vi "Read Power Meter Reverse.vi"(11 "AM-AM in":refnum<class "AM-AM.lvclass">) -> (2 "Power Meter.lvclass":refnum<class "Power Meter.lvclass">, 3 "AM-AM out":refnum<class "AM-AM.lvclass">)   [LabVIEW 2020, in "AM-AM.lvclass"]
uses:
  AM-AM.lvclass
  Instruments/Power Meter/Power Meter.lvclass
  AM-AM.lvclass/AM-AM.ctl
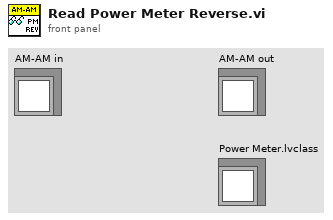
[diagram p1: front panel]
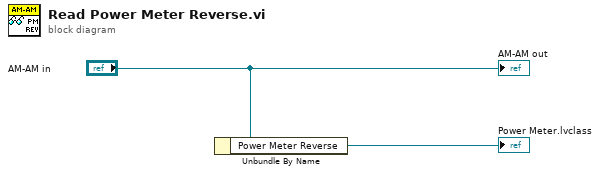
[diagram p0: block diagram]
diagram:
  n1 = Unbundle By Name("AM-AM in") -> ("Power Meter Reverse"=→"Power Meter.lvclass":refnum<class "Power Meter.lvclass">)
  "AM-AM out" <- "AM-AM in"
